vi "Item.vi"(8 "error in (no error)":errorcluster, 10 "Index":i32, 11 "List in":refnum<class "ObjectList.lvclass">) -> (0 "error out":errorcluster, 1 "Item":refnum<class>, 3 "List out":refnum<class "ObjectList.lvclass">)   [LabVIEW 2013, in "LapDog.Collections.v1.Lists.lvlib" / "ObjectList.lvclass"]
doc: "Returns a copy of an item from the list at the given Index. An Index of -1 returns the last item in the list. If no item exists at the given Index error 510201 is returned."
uses:
  ObjectList.lvclass
  ObjectList.lvclass/ObjectList.ctl
  ListImp/ListImp.lvclass
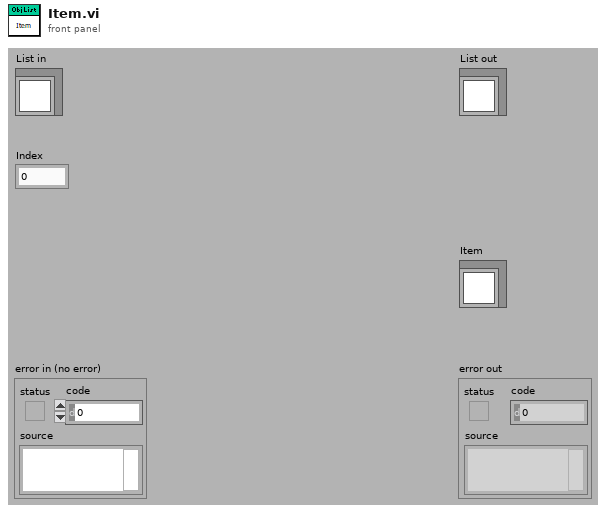
[diagram p1: front panel]
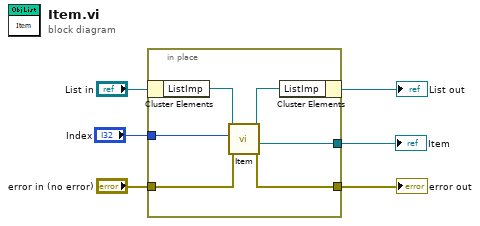
[diagram p0: block diagram]
diagram:
  n1 = in-place {
    in-place-border: "error in (no error)" -> [w12]
    in-place-border: [w11] -> w1
    in-place-border: "Index" -> [w10]
    in-place-border: [w9] -> w4
    n2 = in-place-cluster #1("List in") -> ("ListImp"=w8:refnum<class "ListImp.lvclass">)
    n3 = call-dynamic "Item.vi"("error in (no error)"=w12, "Index"=w10, "ListImp in"=w8) -> ("error out"=w11:errorcluster, "Item"=w9:refnum<class>, "ListImp out"=w7:refnum<class "ListImp.lvclass">)  [unwired: 6 in]
    n4 = in-place-cluster #1("ListImp"=w7) -> (→"List out":refnum<class "ObjectList.lvclass">)
  }
  "error out" <- w1
  "Item" <- w4
